vi "Select Enabled Channel Coefficients.vi"(0 "configured scaling coefficients":cluster{"gain":dbl, "offset":dbl}[](array[cluster]), 5 "selected acq channels to stream":bool[](array[boolean]), 7 "number of selected acq channels to stream":u8) -> (4 "streamed scaling coefficients":cluster{"gain":dbl, "offset":dbl}[](array[cluster]))   [LabVIEW 2015, in "Device Session.lvclass"]
doc: "Selects the scaling coefficients according to the number of channels enabled for acquisition as a nearest power of 2.\n\n<B>Input Parameters</B>\n\n<B>configured scaling coefficients</B> specifies the set of scaling coefficients for all the configured channels.\n\n<B>selected acq channels to stream</B> is a boolean array of the channels enabled for acquisition.\n\n<B>number of selected acq channels to stream</B> is the number of enabled channels rounded up to the nearest power of 2.\n\n<B>Output Parameters</B>\n\n<B>streamed scaling coefficients</B> returns the scaling coefficients selected according to the enabled channels."
uses:
  Device Session.lvclass
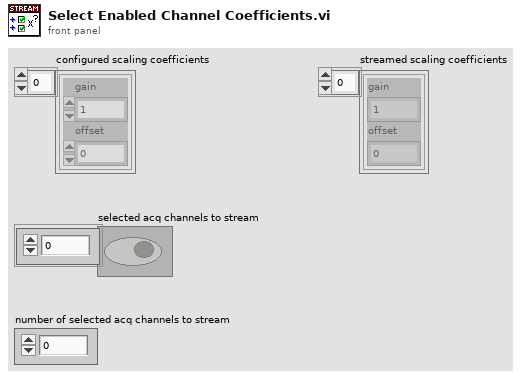
[diagram p1: front panel]
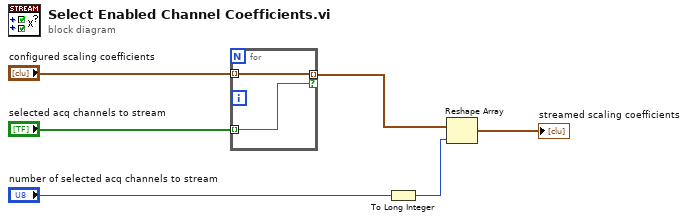
[diagram p0: block diagram]
diagram:
  n1 = for {
    tunnel: "selected acq channels to stream" -> [w8] mode=indexing
    tunnel: [w7] -> w6 mode=indexing if=w8
    tunnel: "configured scaling coefficients" -> [w7] mode=indexing
  }
  n2 = To Long Integer(number="number of selected acq channels to stream") -> (32bit integer=w5:i32)
  n3 = Reshape Array(w6, w5) -> (→"streamed scaling coefficients":cluster{"gain":dbl, "offset":dbl}[])
